vi "Initialize.vi"() -> (0 "error out":errorcluster, 2 "SLAM Out":T1)   [LabVIEW 2009]
uses:
  Controls/SLAM.ctl
  <vilib>/Analysis/Matrix/Datatypes/RealMatrix.ctl
  <vilib>/Analysis/Matrix/NI_Matrix.lvlib
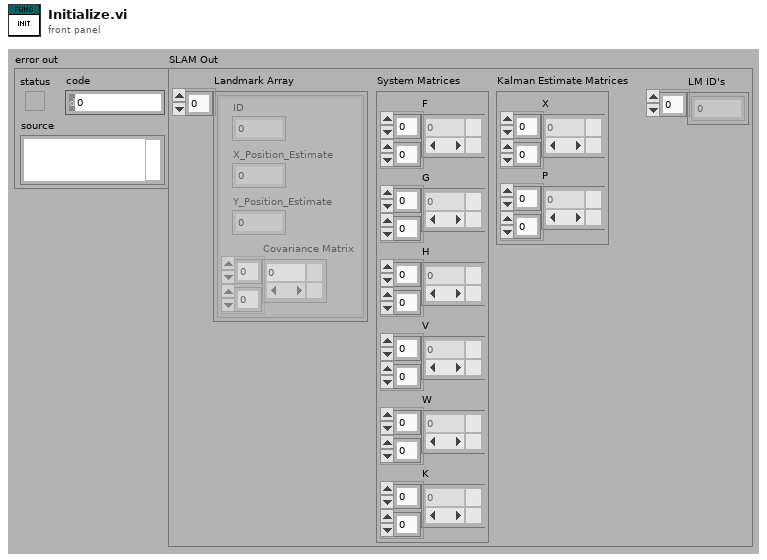
[diagram p1: front panel]
types:
  T1 = typedef "SLAM.ctl" = cluster{"Landmark Array":cluster{"ID":dbl, "X_Position_Estimate":dbl, "Y_Position_Estimate":dbl, "Covariance Matrix":T2}[], "System Matrices":cluster{"F":T2, "G":T2, "H":T2, "V":T2, "W":T2, "K":T2}, "Kalman Estimate Matrices":cluster{"X":T2, "P":T2}, "LM ID's":dbl[]}
  T2 = typedef "NI_Matrix.lvlib/RealMatrix.ctl" = dbl[][]
  T3 = cluster{"F":T2, "G":T2, "H":T2, "V":T2, "W":T2, "K":T2}
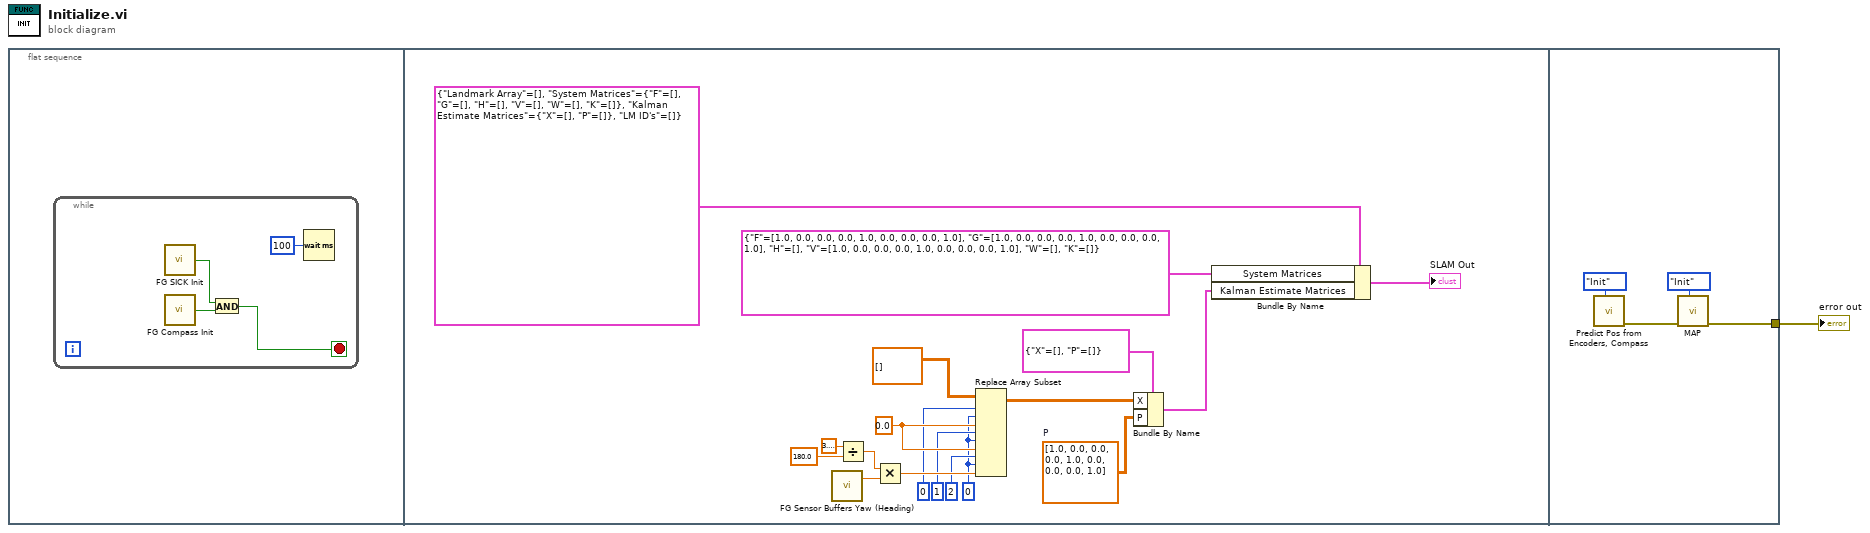
[diagram p0: block diagram]
diagram:
  n1 = flat-sequence {
    tunnel: [w26] -> w1
    frame #0 {
      n2 = while {
        stop <- w3 stop-if-true
        n3 = call "FG SICK Init.vi"() -> ("SICK Init out"=w4:bool)  [unwired: 2 in]
        n4 = call "FG Compass Init.vi"() -> ("Compass Init out"=w5:bool)  [unwired: 2 in]
        n5 = And(x=w4, y=w5) -> (x .and. y?=w3:bool)
        n6 = Wait (ms)(milliseconds to wait=u32 100) -> ()  [unwired: 1 out]
      }
    }
    frame #1 {
      w20 = T2 [[1.0, 0.0, 0.0], [0.0, 1.0, 0.0], [0.0, 0.0, 1.0]]  # P
      w18 = 0.0 ("new element/submatrix")
      w10 = 0 ("disabled index (col)")
      n7 = call "FG Sensor Buffers Yaw (Heading).vi"() -> ("Yaw Buffer Out"=w13:dbl)  [unwired: 3 in]
      n8 = Divide(x=3.141592653589793, y=180.0) -> (x/y=w14:dbl)
      n9 = Multiply(x=w14, y=w13) -> (x*y=w17:dbl)
      n10 = Replace Array Subset(array=T2 [] ("matrix"), new element #1=w18, index (row) #1=0 ("disabled index (row)"), index (col) #1=w10, new element #2=w18, index (row) #2=1 ("disabled index (row)"), index (col) #2=w10, new element #3=w17, index (row) #3=2 ("disabled index (row)"), index (col) #3=w10) -> (w21:T2)
      n11 = Bundle By Name(cluster=cluster{"X":T2, "P":T2} {"X"=[], "P"=[]} ("Kalman Estimate Matrices"), "X"=w21, "P"=w20) -> (w8:cluster{"X":T2, "P":T2})
      n12 = Bundle By Name(cluster=T1 {"Landmark Array"=[], "System Matrices"={"F"=[], "G"=[], "H"=[], "V"=[], "W"=[], "K"=[]}, "Kalman Estimate Matrices"={"X"=[], "P"=[]}, "LM ID's"=[]} ("SLAM"), "System Matrices"=T3 {"F"=[[1.0, 0.0, 0.0], [0.0, 1.0, 0.0], [0.0, 0.0, 1.0]], "G"=[[1.0, 0.0, 0.0], [0.0, 1.0, 0.0], [0.0, 0.0, 1.0]], "H"=[], "V"=[[1.0, 0.0, 0.0], [0.0, 1.0, 0.0], [0.0, 0.0, 1.0]], "W"=[], "K"=[]}, "Kalman Estimate Matrices"=w8) -> (→"SLAM Out":T1)
    }
    frame #2 {
      n13 = call "Predict Pos from Encoders, Compass.vi"("Cmd"=enum16{"Init", "Run"}."Init") -> ("error out"=w25:errorcluster)  [unwired: 9 in, 1 out]
      n14 = call "MAP.vi"("Cmd"=enum16{"Init", "Run"}."Init", "error in (no error)"=w25) -> ("error out"=w26:errorcluster)  [unwired: 6 in, 3 out]
    }
  }
  "error out" <- w1
